vi "Init.vi"(8 "error in":errorcluster, 10 "OD Entry":refnum<class "OD Entry.lvclass">, 11 "Transmit PDO in":refnum<class "TX PDO Communication Parameter.lvclass">) -> (0 "error out":errorcluster, 3 "Transmit PDO out":refnum<class "TX PDO Communication Parameter.lvclass">)   [LabVIEW 2024, in "PDO Grid.lvlib" / "TX PDO Communication Parameter.lvclass"]
uses:
  TX PDO Communication Parameter.lvclass
  Core/OD Entry/OD Entry.lvclass
  TX PDO Communication Parameter.lvclass/TX PDO Communication Parameter.ctl
  Core/Value/Value.lvclass
  Core/PDO Communication Parameter/PDO Communication Parameter.lvclass
  D:/git/EDS-File-Viewer/source/Core/PDO Communication Parameter/PDO Communication Parameter.lvclass
  D:/git/EDS-File-Viewer/source/TPDO Communication Parameter/TX PDO Communication Parameter.lvclass
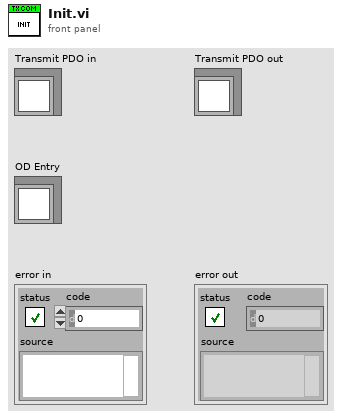
[diagram p1: front panel]
types:
  T1 = enum16{"ro", "wo", "rw", "rwr", "rww", "const", "UNKNOWN"}
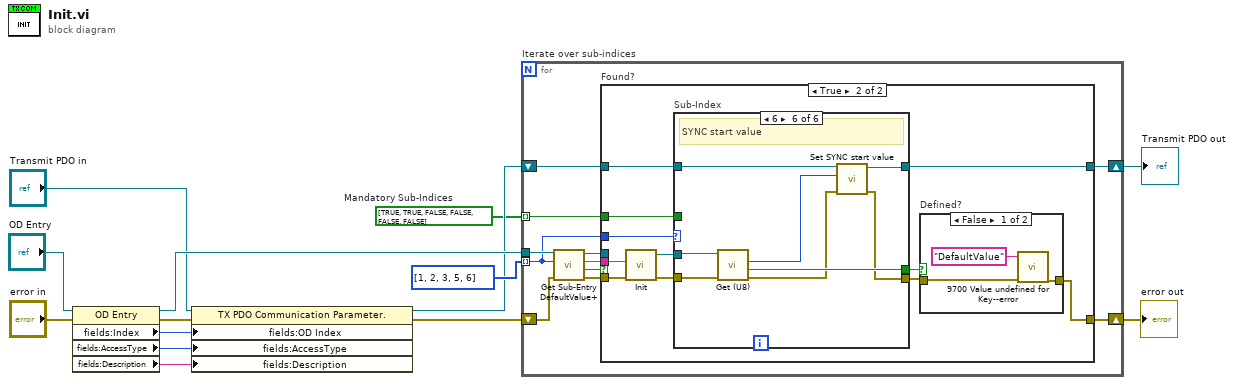
[diagram p0: block diagram]
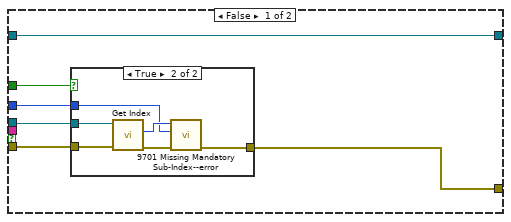
[diagram p2: hidden frame]
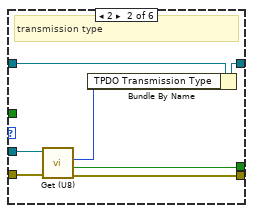
[diagram p5: hidden frame]
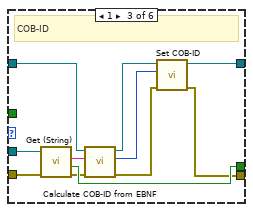
[diagram p6: hidden frame]
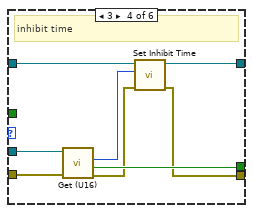
[diagram p7: hidden frame]
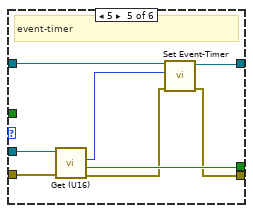
[diagram p8: hidden frame]
diagram:
  w1 = bool[] [TRUE, TRUE, FALSE, FALSE, FALSE, FALSE]  # Mandatory Sub-Indices
  n1 = property class="OD Entry"(reference="OD Entry", error in="error in") -> (reference out=w8:refnum<class "OD Entry.lvclass">, error out=w10:errorcluster, "fields:Index"=w5:u16, "fields:AccessType"=w4:T1, "fields:Description"=w3:string)
  n2 = property class="TX PDO Communication Parameter."(reference="Transmit PDO in", error in=w10, "fields:OD Index"=w5, "fields:AccessType"=w4, "fields:Description"=w3) -> (reference out=w6:refnum<class "TX PDO Communication Parameter.lvclass">, error out=w7:errorcluster)
  n3 = for "Iterate over sub-indices" {
    tunnel: u16[] [1, 2, 3, 5, 6] -> [w20] mode=indexing
    shift-right: [w24] -> w11
    shift-left: w6 -> [w25]
    shift-right: [w23] -> w12
    shift-left: w7 -> [w19]
    tunnel: w8 -> [w22]
    tunnel: w1 -> [w15] mode=indexing
    n4 = call "Get Sub-Entry DefaultValue+.vi"("Error In"=w19, "Sub-Index"=w20, "reference in"=w22) -> ("Error Out"=w18:errorcluster, "Found?"=w17:bool, "DefaultValue"=w16:string, "reference out"=w21:refnum<class "OD Entry.lvclass">)  [unwired: 5 in]
    n5 = case "Found?" shown="True" w17 {
      tunnel: w25 -> [w27 w49]
      tunnel: [w27 w48] -> w24
      tunnel: [w28 w41] -> w23
      tunnel: w21 -> [w30 _]
      tunnel: w20 -> [w29 w47]
      tunnel: w18 -> [w31 w46]
      tunnel: w16 -> [_ w40]
      tunnel: w15 -> [w26 w39]
      frame False {
        n6 = case shown="True" w26 {
          tunnel: w31 -> [w32 w37]
          tunnel: w30 -> [_ w36]
          tunnel: w29 -> [_ w33]
          tunnel: [w32 w35] -> w28
          frame False {
          }
          frame True {
            n7 = call "Get Index.vi"("Error In"=w37, "reference in"=w36) -> ("Error Out"=w38:errorcluster, "Index"=w34:u16)  [unwired: 7 in, 1 out]
            n8 = call "9701 Missing Mandatory Sub-Index--error.vi"("error in"=w38, "Sub-Index"=w33, "Index"=w34) -> ("error out"=w35:errorcluster)  [unwired: 8 in]
          }
        }
      }
      frame True {
        n9 = call "Init.vi"("error in"=w46, "Value"=w40) -> ("error out"=w45:errorcluster, "Value out"=w44:refnum<class "Value.lvclass">)  [unwired: 8 in]
        n10 = case "Sub-Index" shown="6" w47 {
          tunnel: w49 -> [w51 w58 w64 w73 w81 w89]
          tunnel: [w51 w57 w62 w72 w80 w88] -> w48
          tunnel: w45 -> [w50 w55 w66 w75 w84 w92]
          tunnel: w44 -> [_ w54 w68 w76 w83 w91]
          tunnel: [_ w53 w67 w74 w82 w90] -> w43
          tunnel: [w50 w52 w59 w70 w77 w85] -> w42
          tunnel: w39 -> [_ _ _ _ _ _]
          frame Default {
            # "can't be reached"
          }
          frame 2 {
            # "transmission type"
            n11 = call "Get (U8).vi"("error in"=w55, "Value in"=w54) -> ("error out"=w52:errorcluster, "Defined?"=w53:bool, "Value"=w56:u8)  [unwired: 6 in, 1 out]
            n12 = Bundle By Name(cluster=w58, "TPDO Transmission Type"=w56) -> (w57:refnum<class "TX PDO Communication Parameter.lvclass">)
          }
          frame 1 {
            # "COB-ID"
            n13 = call "Get (String).vi"("Value in"=w68) -> ("Defined?"=w67:bool, "Value"=w65:string)  [unwired: 8 in, 1 out]
            n14 = call "Calculate COB-ID from EBNF.vi"("error in"=w66, "ENBF"=w65, "Transmit PDO in"=w64) -> ("error out"=w60:errorcluster, "COB-ID"=w61:u32, "Transmit PDO out"=w63:refnum<class "TX PDO Communication Parameter.lvclass">)  [unwired: 6 in]
            n15 = call "Set COB-ID.vi"("error in (no error)"=w60, "COB-ID"=w61, "PDO Communication Parameter in"=w63) -> ("error out"=w59:errorcluster, "PDO Communication Parameter out"=w62:refnum<class "TX PDO Communication Parameter.lvclass">)  [unwired: 7 in]
          }
          frame 3 {
            # "inhibit time"
            n16 = call "Get (U16).vi"("error in"=w75, "Value in"=w76) -> ("error out"=w71:errorcluster, "Defined?"=w74:bool, "Value"=w69:u16)  [unwired: 6 in, 1 out]
            n17 = call "Set Inhibit Time.vi"("error in"=w71, "Inhibit Time"=w69, "PDO Communication Parameter in"=w73) -> ("error out"=w70:errorcluster, "PDO Communication Parameter out"=w72:refnum<class "TX PDO Communication Parameter.lvclass">)  [unwired: 7 in]
          }
          frame 5 {
            # "event-timer"
            n18 = call "Get (U16).vi"("error in"=w84, "Value in"=w83) -> ("error out"=w78:errorcluster, "Defined?"=w82:bool, "Value"=w79:u16)  [unwired: 6 in, 1 out]
            n19 = call "Set Event-Timer.vi"("error in (no error)"=w78, "Event-Timer"=w79, "PDO Communication Parameter in"=w81) -> ("error out"=w77:errorcluster, "PDO Communication Parameter out"=w80:refnum<class "TX PDO Communication Parameter.lvclass">)  [unwired: 7 in]
          }
          frame 6 {
            # "SYNC start value"
            n20 = call "Get (U8).vi"("error in"=w92, "Value in"=w91) -> ("error out"=w86:errorcluster, "Defined?"=w90:bool, "Value"=w87:u8)  [unwired: 6 in, 1 out]
            n21 = call "Set SYNC start value.vi"("error in (no error)"=w86, "SYNC start value"=w87, "PDO Communication Parameter in"=w89) -> ("error out"=w85:errorcluster, "PDO Communication Parameter out"=w88:refnum<class "TX PDO Communication Parameter.lvclass">)  [unwired: 7 in]
          }
        }
        n22 = case "Defined?" shown="False" w43 {
          tunnel: w42 -> [w94 w96]
          tunnel: [w95 w96] -> w41
          frame False {
            n23 = call "9700 Value undefined for Key--error.vi"("error in"=w94, "Argument"="DefaultValue" ("key")) -> ("error out"=w95:errorcluster)  [unwired: 9 in]
          }
          frame True {
          }
        }
      }
    }
  }
  "Transmit PDO out" <- w11
  "error out" <- w12
